vi "SubModule.vi"() -> ()   [LabVIEW 2020]
uses:
  <userlib>/_NEVSTOP/JKI State Machine++/_Support/JKISMQ/_Obtain JKISMQ.vi
  <userlib>/_NEVSTOP/JKI State Machine++/_Support/FGV-BroadcastRegistry/Cache-Broadcast Registry Search Result.vi
  <userlib>/_NEVSTOP/JKI State Machine++/_Support/JKISMQ/_Create Resp Queue.vi
  <userlib>/_NEVSTOP/JKI State Machine++/_Support/JKISMQ/_Unlock JKISMQ.vi
  <userlib>/_NEVSTOP/JKI State Machine++/_Support/JKISMQ/_Lock State JKISMQ.vi
  <userlib>/_NEVSTOP/JKI State Machine++/_Support/JKISMQ/_Release JKISMQ.vi
  <userlib>/_NEVSTOP/JKI State Machine++/_Support/JKISMQ/_Input Name to JKISM Mode.vi
  <userlib>/_NEVSTOP/JKI State Machine++/Utility/uuid.vi
  <userlib>/_NEVSTOP/JKI State Machine++/_Support/FGV-BroadcastRegistry/global-JKISMQ FGV Change Flag.vi
  <userlib>/_NEVSTOP/JKI State Machine++/_Support/JKISMQ/_JKISMQFGV.vi
  <userlib>/_NEVSTOP/JKI State Machine++/_Support/GlobalEvent/FGV-GlobalEventRef.vi
  <userlib>/_NEVSTOP/JKI State Machine++/_Support/JKISMQ/_Dequeue JKISMQ.vi
  <userlib>/_NEVSTOP/JKI State Machine++/_Support/JKISMQ/_Enqueue JKISMQ.vi
  <userlib>/_NEVSTOP/JKI State Machine++/_Support/FGV-BroadcastRegistry/global-Broadcast Cache Change Flag.vi
  <userlib>/_NEVSTOP/JKI State Machine++/_Support/FGV-BroadcastRegistry/FGV-BroadcastRegistry.vi
  <userlib>/_NEVSTOP/JKI State Machine++/JKI State Machine++.lvlib
panel:
  out "State History":string
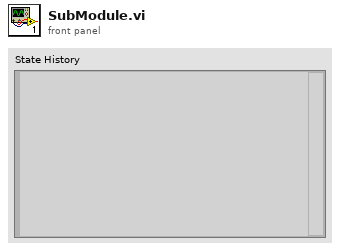
[diagram p1: front panel]
types:
  T1 = enum32{"Invalid", "Standard", "Closed", "Hidden", "Minimized", "Maximized"}
  T2 = enum32{"invalid app kind", "Development System", "Run Time System", "Student Edition", "Embedded LabVIEW", "Evaluation", "Custom"}
  T3 = cluster{"Core":cluster{"Current VI Reference":refnum<vi>, "Close Panel on Exit?":bool}, "Your Boolean data":bool, "Your string data":string}
  T4 = cluster{"Current VI Reference":refnum<vi>, "Close Panel on Exit?":bool}
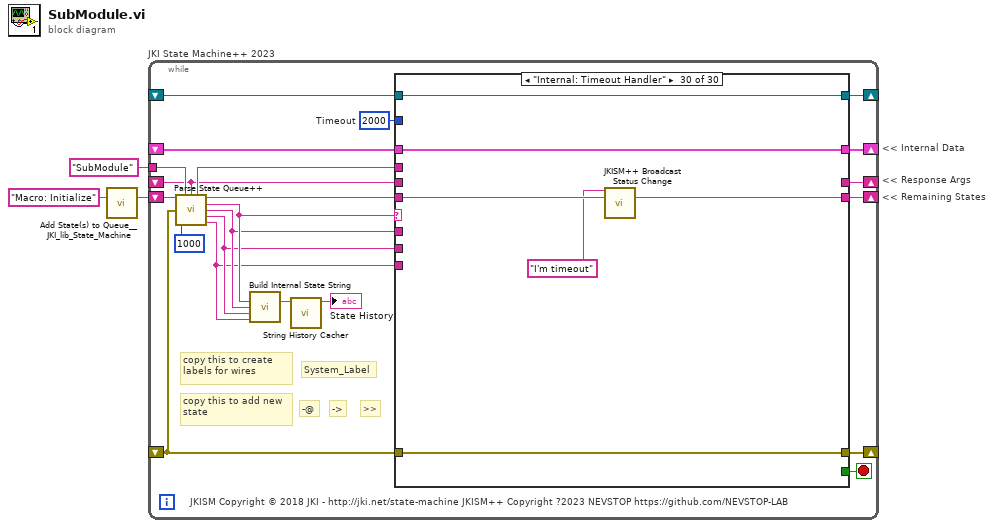
[diagram p0: block diagram]
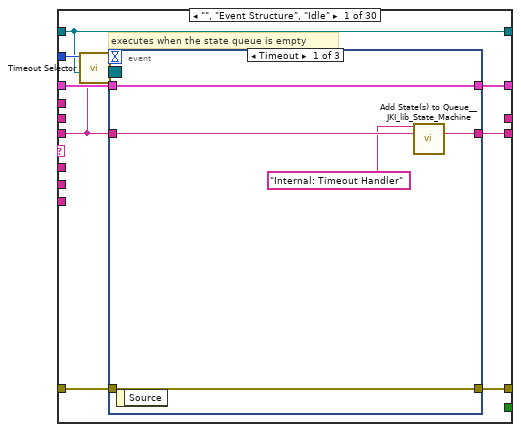
[diagram p2: hidden frame]
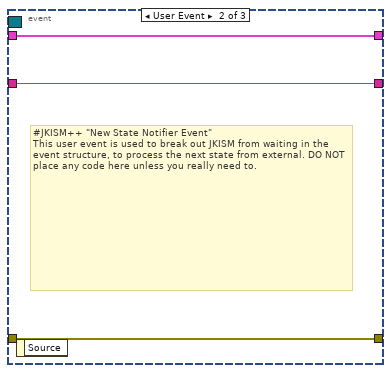
[diagram p3: hidden frame]
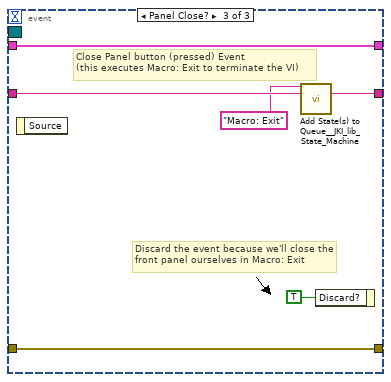
[diagram p4: hidden frame]
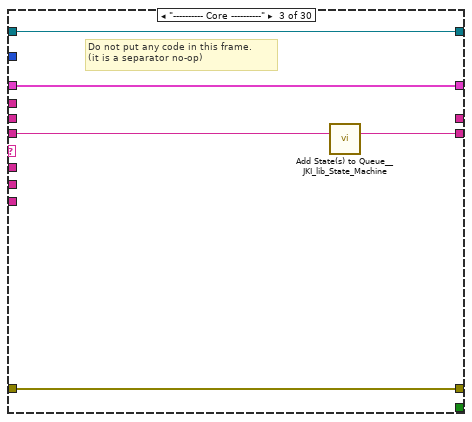
[diagram p6: hidden frame]
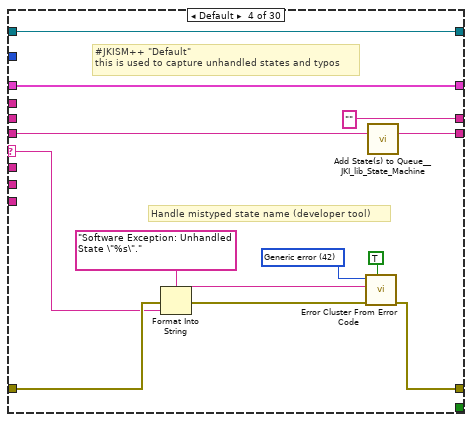
[diagram p7: hidden frame]
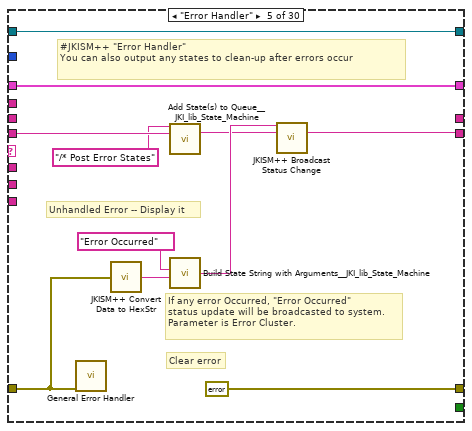
[diagram p8: hidden frame]
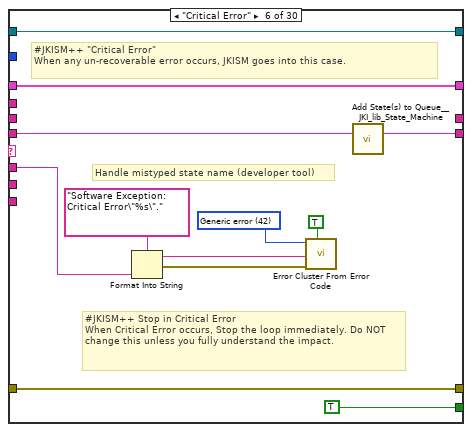
[diagram p9: hidden frame]
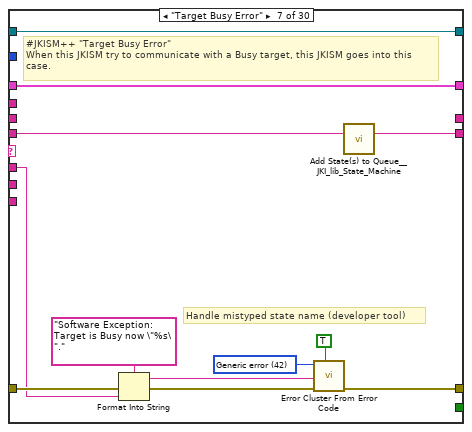
[diagram p10: hidden frame]
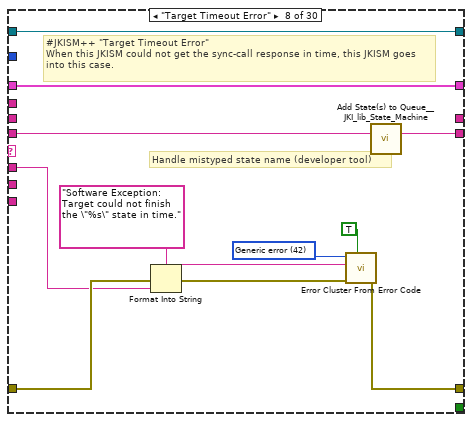
[diagram p11: hidden frame]
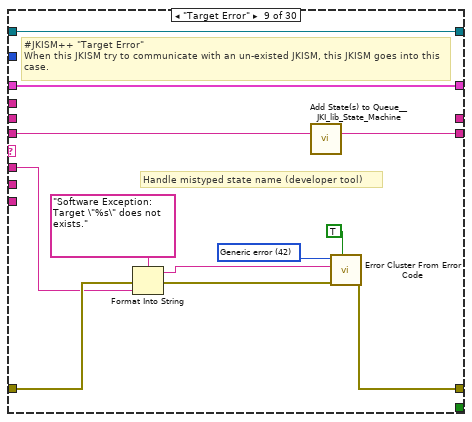
[diagram p12: hidden frame]
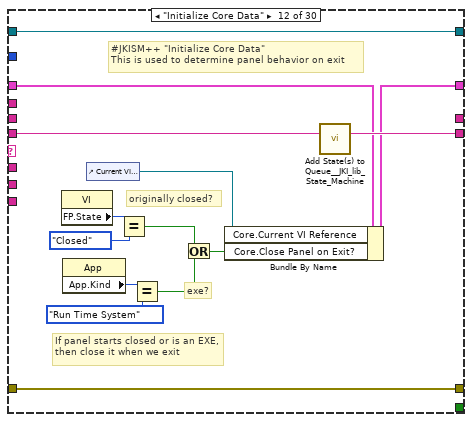
[diagram p15: hidden frame]
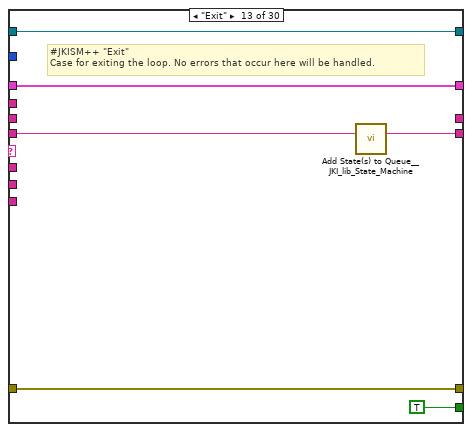
[diagram p16: hidden frame]
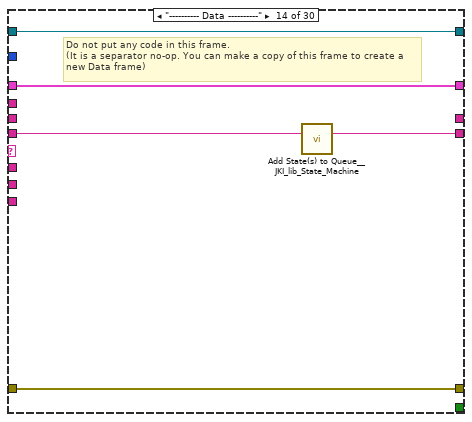
[diagram p17: hidden frame]
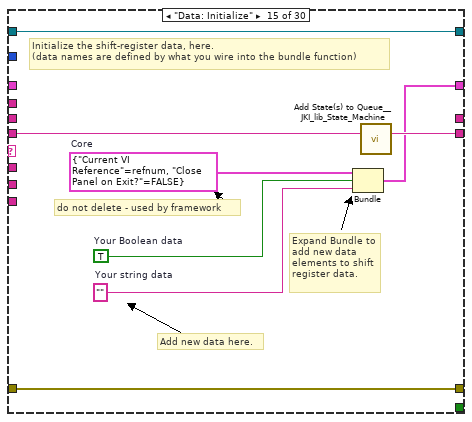
[diagram p18: hidden frame]
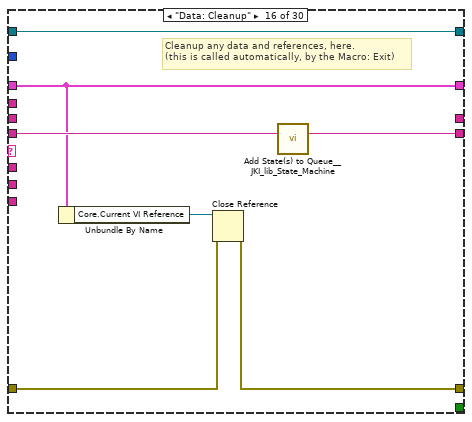
[diagram p19: hidden frame]
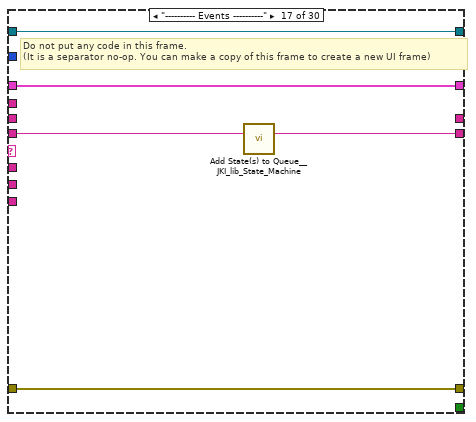
[diagram p20: hidden frame]
diagram:
  # "<< Internal Data"
  # "<< Response Args"
  # "<< Remaining States"
  n1 = call <vilib>:"Add State(s) to Queue__JKI_lib_State_Machine.vi"("State(s) in (\"\")"="Macro: Initialize") -> ("States Out"=w1:string)  [unwired: 14 in]
  n2 = while "JKI State Machine++ 2023" {
    shift-right: [w20] -> _
    shift-left: _ -> [w19]
    shift-right: [w23] -> _
    shift-left: _ -> [w17]
    shift-right: [w22] -> _
    shift-left: w1 -> [w24]
    tunnel: "SubModule" ("Name(\"\" to use uuid)") -> [w12]
    shift-right: [w15] -> _
    shift-left: _ -> [w4]
    shift-right: [w14] -> _
    shift-left: _ -> [w13]
    stop <- w21 stop-if-true
    w18 = 2000  # Timeout
    # "JKISM Copyright © 2018 JKI - http://jki.net/state-machine JKISM++ Copyright ?2023 NEVSTOP https://github.com/NEVSTOP-LAB"
    # "copy this to add new state"
    # ">>"
    # "->"
    # "-@"
    # "copy this to create labels for wires"
    # "System_Label"
    n3 = call <userlib>:"Parse State Queue++.vi"("State Queue"=w24, "Name(\"\" to use uuid)"=w12, "Response Arguments"=w4, "Error In (no error)"=w17, "Response Timeout(5000ms)"=1000 ("Response Timeout(1000ms)")) -> ("Name Used"=w5:string, "Remaining States"=w25:string, "Current State"=w9:string, "Arguments"=w8:string, "Argument - State"=w7:string, "From Who"=w6:string)  [unwired: 5 in]
    n4 = call <userlib>:"Build Internal State String.vi"("State"=w9, "Arguments (\"\")"=w8, "Arg-State (\"\")"=w7, "Source (\"\")"=w6) -> ("State with Arguments"=w10:string)  [unwired: 11 in]
    n5 = call <userlib>:"String History Cacher.vi"("String"=w10) -> ("String Cache"=→"State History":string)  [unwired: 10 in]
    n6 = case shown="\"Internal: Timeout Handler\"" w9 {
      selector: w9 -> [_ _ _ w60 _ _ _ _ _ _ _ _ _ _ _ _ _ _ _ _ _ _ _ _ _ _ _ _ _ _]
      tunnel: w25 -> [w26 w51 w57 w64 w81 w91 w94 w111 w123 w132 w136 w151 w157 w162 w170 w177 w182 w189 w193 w199 w204 w211 w227 w297 w303 w314 w317 w324 w328 w331]
      tunnel: w8 -> [_ _ _ _ _ w84 w96 w107 w119 _ _ _ _ _ _ _ _ _ _ _ _ w206 w221 _ _ _ _ w319 _ _]
      tunnel: w19 -> [w33 w50 w54 w62 w79 w92 w98 w109 w121 w131 w135 w144 w155 w159 _ w172 w179 w188 w192 w196 w202 w209 w223 w294 w300 w311 w316 w323 w327 w334]
      tunnel: [w32 w52 w55 w66 errorcluster {"status"=FALSE, "code"=0, "source"=""} ("error out") w93 w101 w113 w125 w133 w137 w148 w154 w160 w167 w173 w180 w183 w191 w197 w201 w207 w224 w295 w301 w312 w318 w325 w329 w335] -> w23
      tunnel: w17 -> [w31 w52 w55 w65 w71 w93 w100 w112 w124 w133 w137 w148 w154 w160 w167 w174 w180 _ w194 w197 w201 w208 w225 w295 w301 w312 w318 w325 w329 w335]
      tunnel: [w34 w51 w56 w63 w72 w90 w99 w110 w122 w132 w136 w150 w156 w161 w169 w176 w181 w189 w193 w198 w203 w210 w226 w296 w302 w313 w317 w324 w328 w332] -> w22
      tunnel: [_ _ _ _ _ TRUE _ _ _ _ _ _ TRUE _ _ _ _ _ _ _ _ _ _ _ _ _ _ _ _ _] -> w21
      tunnel: [w30 w50 w54 w62 w79 w92 w98 w109 w121 w131 w135 w149 w155 w159 w168 w172 w179 w188 w192 w196 w202 w209 w223 w294 w300 w311 w316 w323 w327 w334] -> w20
      tunnel: w18 -> [w29 _ _ _ _ _ _ _ _ _ _ _ _ _ _ _ _ _ _ _ _ _ _ _ _ _ _ _ _ _]
      tunnel: w6 -> [_ _ _ _ _ _ _ _ _ _ _ _ _ _ _ _ _ _ _ _ _ _ _ _ _ _ _ _ _ _]
      tunnel: w7 -> [_ _ _ _ _ _ _ _ _ _ _ _ _ _ _ _ _ _ _ _ _ _ _ _ _ _ _ _ _ _]
      tunnel: [_ _ _ "" _ _ _ _ _ _ _ _ _ _ _ _ _ _ _ _ _ _ _ _ _ _ _ w320 _ _] -> w15
      tunnel: [w28 w49 w53 w58 w77 w82 w95 w106 w118 w130 w134 w138 w152 w158 w163 w171 w178 w187 w190 w195 w200 w205 w220 w293 w298 w304 w315 w322 w326 w333] -> w14
      tunnel: w13 -> [w28 w49 w53 w58 w77 w82 w95 w106 w118 w130 w134 w138 w152 w158 w163 w171 w178 _ w190 w195 w200 w205 w220 w293 w298 w304 w315 w322 w326 w333]
      tunnel: w5 -> [_ _ _ _ _ _ _ _ _ _ _ _ _ _ _ _ _ w186 _ _ _ _ _ _ _ _ _ _ _ _]
      tunnel: w4 -> [_ _ _ _ _ _ _ _ _ _ _ _ _ _ _ _ _ _ _ _ _ _ _ _ _ _ _ _ _ _]
      frame "", "Event Structure", "Idle" {
        # "executes when the state queue is empty"
        n7 = call <userlib>:"Timeout Selector.vi"("Remaining States"=w26, "Timeout Expected"=w29) -> ("Timeout"=w27:i32)  [unwired: 5 in]
        n8 = event shown="[0] Timeout" {
          selector: w28 -> [_ _ _]
          dyn-events: _ -> [_ _ _]
          timeout: w27 -> [_ _ _]
          tunnel: w26 -> [w39 w41 w48]
          tunnel: [w38 w41 w47] -> w34
          tunnel: w33 -> [w36 w42 w45]
          tunnel: [w37 w40 w46] -> w32
          tunnel: w31 -> [w37 w40 w46]
          tunnel: [w36 w42 w45] -> w30
          event Timeout {
            n9 = event-data() -> ()  [unwired: 1 in, 1 out]
            n10 = call <vilib>:"Add State(s) to Queue__JKI_lib_State_Machine.vi"("State(s) in Front (\"\")"="Internal: Timeout Handler" ("State(s) in Front (\"\")"), "State(s) in (\"\")"=w39) -> ("States Out"=w38:string)  [unwired: 13 in]
          }
          event User Event {
            # "#JKISM++ \"New State Notifier Event\"\nThis user event is used to break out JKISM from waiting in the event structure, to process the next state from external. DO NOT place any code here unless you really need to."
            n11 = event-data() -> ()  [unwired: 1 in, 1 out]
          }
          event Panel Close? {
            # "Discard the event because we'll close the front panel ourselves in Macro: Exit"
            # "Close Panel button (pressed) Event\n(this executes Macro: Exit to terminate the VI)"
            n12 = event-data() -> ()  [unwired: 1 in, 1 out]
            n13 = call <vilib>:"Add State(s) to Queue__JKI_lib_State_Machine.vi"("State(s) in Front (\"\")"="Macro: Exit", "State(s) in (\"\")"=w48) -> ("States Out"=w47:string)  [unwired: 13 in]
            n14 = event-data("Discard?"=TRUE) -> ()  [unwired: 1 in, 1 out]
          }
        }
      }
      frame "JKISM++ Documentation" {
        # "#JKISM++ \"Documentation\"\nCase for holding JKISM++ Documenation"
      }
      frame "---------- Core ----------" {
        # "Do not put any code in this frame.\n(it is a separator no-op)"
        n15 = call <vilib>:"Add State(s) to Queue__JKI_lib_State_Machine.vi"("State(s) in (\"\")"=w57) -> ("States Out"=w56:string)  [unwired: 14 in]
      }
      frame Default {
        w69 = 42 items=["No error", "Argument error", "Memory is full", "Out of zone", "End of file", "File already open", "Generic file I/O error", "File not found", "File permission error", "Disk is full", "Duplicate path", "Too many files open", "System feature not enabled", "Resource file not found", "Cannot add resource", "Resource not found", "Image not found", "Image memory error", "Pen does not exist", "Config type invalid", "Config token not found", "Config parse error", "Config memory error", "Bad external code format", "Bad external code offset", "External code not present", "Null window", "Destroy window error", "Null menu", "Print aborted", "Bad print record", "Print driver error", "Windows error during printing", "Memory error during printing", "Print dialog error", "Generic print error", "Invalid device refnum", "Device not found", "Device parameter error", "Device unit error", "Cannot open device", "Device call aborted", "Generic error", "Cancelled by user", "Object ID too low", "Object ID too high", "Object not in heap", "Unknown heap", "Unknown object (invalid DefProc)", "Unknown object (DefProc not in table)", "Message out of range", "Invalid (null) method", "Unknown message", "Manager call not supported", "Bad address", "Network operation in progress", "Network operation timed out", "Connection is busy", "Network attribute not supported", "Network error", "Address in use", "System out of memory", "Connection aborted", "Connection refused", "Not connected", "Already connected", "Connection closed", "Initialization error (interapplication manager)", "Bad occurrence", "Wait on unbound occurrence handler", "Occurrence queue overflow", "Datalog type conflict", "Unused", "Unrecognized type (interapplication manager)", "Memory corrupt", "Failed to make temporary DLL", "Old CIN version", "Drag socket not found", "Failed to load drop-object", "Failed to register OLE object", "Failed to release OLE object", "Format specifier type mismatch", "Unknown format specifier", "Too few format specifiers", "Too many format specifiers", "Scan failed", "Newer CIN version", "Error converting to variant", "Runtime menu error", "Password tampered", "Variant attribute not found", "Incompatible variant data type", "Event data is not available", "Event Store is not present", "Occurrence is not found", "Event Queue is not created", "Event info is not available", "Refnum passed is NULL", "Error retrieving Class GUID", "Error retrieving CoClass GUID", "Error retrieving TypeLib GUID.", "Bad built application magic bytes.", "Specific driver is different from the specific driver associated with the Logical Name.", "There is no session opened to the class driver.", "Max Error", "MAX - Error with config objects", "MAX - Error loading configuration", "MAX - Group not supported"]
        # "#JKISM++ \"Default\"\nthis is used to capture unhandled states and typos"
        # "Handle mistyped state name (developer tool)"
        n16 = Format Into String(format string="Software Exception: Unhandled State \"%s\"." ("message"), error in=w65, w60) -> (resulting string=w68:string, error out=w67:errorcluster)  [unwired: 1 in]
        n17 = call <vilib>:"Error Cluster From Error Code.vi"("show call chain? (False)"=TRUE, "error in (no error)"=w67, "error message (\"\")"=w68, "error code (0)"=w69) -> ("error out"=w66:errorcluster)  [unwired: 5 in]
        n18 = call <vilib>:"Add State(s) to Queue__JKI_lib_State_Machine.vi"("State(s) in (\"\")"=w64) -> ("States Out"=w63:string)  [unwired: 14 in]
      }
      frame "Error Handler" {
        # "#JKISM++ \"Error Handler\"\nYou can also output any states to clean-up after errors occur"
        # "If any error Occurred, \"Error Occurred\" \nstatus update will be broadcasted to system.\nParameter is Error Cluster."
        # "Unhandled Error -- Display it"
        # "Clear error"
        n19 = call <vilib>:"General Error Handler.vi"("error in (no error)"=w71) -> ()  [unwired: 10 in, 5 out]
        n20 = call <userlib>:"JKISM++ Convert Data to HexStr.vi"("Variant"=w71) -> ("HEX String (0-9,A-F)"=w75:string)  [unwired: 8 in]
        n21 = call <vilib>:"Add State(s) to Queue__JKI_lib_State_Machine.vi"("State(s) in Front (\"\")"="/* Post Error States", "State(s) in (\"\")"=w81) -> ("States Out"=w73:string)  [unwired: 13 in]
        n22 = call <vilib>:"Build State String with Arguments__JKI_lib_State_Machine.vi"("Arguments (\"\")"=w75, "State"="Error Occurred" ("Status with Arguments")) -> ("State with Arguments"=w74:string)  [unwired: 4 in]
        n23 = call <userlib>:"JKISM++ Broadcast Status Change.vi"("Status with Arguments"=w74, "State Queue"=w73) -> ("Remaining States"=w72:string)  [unwired: 13 in]
      }
      frame "Critical Error" {
        w88 = 42 items=["No error", "Argument error", "Memory is full", "Out of zone", "End of file", "File already open", "Generic file I/O error", "File not found", "File permission error", "Disk is full", "Duplicate path", "Too many files open", "System feature not enabled", "Resource file not found", "Cannot add resource", "Resource not found", "Image not found", "Image memory error", "Pen does not exist", "Config type invalid", "Config token not found", "Config parse error", "Config memory error", "Bad external code format", "Bad external code offset", "External code not present", "Null window", "Destroy window error", "Null menu", "Print aborted", "Bad print record", "Print driver error", "Windows error during printing", "Memory error during printing", "Print dialog error", "Generic print error", "Invalid device refnum", "Device not found", "Device parameter error", "Device unit error", "Cannot open device", "Device call aborted", "Generic error", "Cancelled by user", "Object ID too low", "Object ID too high", "Object not in heap", "Unknown heap", "Unknown object (invalid DefProc)", "Unknown object (DefProc not in table)", "Message out of range", "Invalid (null) method", "Unknown message", "Manager call not supported", "Bad address", "Network operation in progress", "Network operation timed out", "Connection is busy", "Network attribute not supported", "Network error", "Address in use", "System out of memory", "Connection aborted", "Connection refused", "Not connected", "Already connected", "Connection closed", "Initialization error (interapplication manager)", "Bad occurrence", "Wait on unbound occurrence handler", "Occurrence queue overflow", "Datalog type conflict", "Unused", "Unrecognized type (interapplication manager)", "Memory corrupt", "Failed to make temporary DLL", "Old CIN version", "Drag socket not found", "Failed to load drop-object", "Failed to register OLE object", "Failed to release OLE object", "Format specifier type mismatch", "Unknown format specifier", "Too few format specifiers", "Too many format specifiers", "Scan failed", "Newer CIN version", "Error converting to variant", "Runtime menu error", "Password tampered", "Variant attribute not found", "Incompatible variant data type", "Event data is not available", "Event Store is not present", "Occurrence is not found", "Event Queue is not created", "Event info is not available", "Refnum passed is NULL", "Error retrieving Class GUID", "Error retrieving CoClass GUID", "Error retrieving TypeLib GUID.", "Bad built application magic bytes.", "Specific driver is different from the specific driver associated with the Logical Name.", "There is no session opened to the class driver.", "Max Error", "MAX - Error with config objects", "MAX - Error loading configuration", "MAX - Group not supported"]
        # "#JKISM++ Stop in Critical Error\nWhen Critical Error occurs, Stop the loop immediately. Do NOT change this unless you fully understand the impact."
        # "#JKISM++ \"Critical Error\"\nWhen any un-recoverable error occurs, JKISM goes into this case."
        # "Handle mistyped state name (developer tool)"
        n24 = Format Into String(format string="Software Exception: Critical Error\"%s\"." ("message"), w84) -> (resulting string=w87:string, error out=w86:errorcluster)  [unwired: 2 in]
        n25 = call <vilib>:"Error Cluster From Error Code.vi"("show call chain? (False)"=TRUE, "error in (no error)"=w86, "error message (\"\")"=w87, "error code (0)"=w88) -> ()  [unwired: 5 in, 1 out]
        n26 = call <vilib>:"Add State(s) to Queue__JKI_lib_State_Machine.vi"("State(s) in (\"\")"=w91) -> ("States Out"=w90:string)  [unwired: 14 in]
      }
      frame "Target Busy Error" {
        w104 = 42 items=["No error", "Argument error", "Memory is full", "Out of zone", "End of file", "File already open", "Generic file I/O error", "File not found", "File permission error", "Disk is full", "Duplicate path", "Too many files open", "System feature not enabled", "Resource file not found", "Cannot add resource", "Resource not found", "Image not found", "Image memory error", "Pen does not exist", "Config type invalid", "Config token not found", "Config parse error", "Config memory error", "Bad external code format", "Bad external code offset", "External code not present", "Null window", "Destroy window error", "Null menu", "Print aborted", "Bad print record", "Print driver error", "Windows error during printing", "Memory error during printing", "Print dialog error", "Generic print error", "Invalid device refnum", "Device not found", "Device parameter error", "Device unit error", "Cannot open device", "Device call aborted", "Generic error", "Cancelled by user", "Object ID too low", "Object ID too high", "Object not in heap", "Unknown heap", "Unknown object (invalid DefProc)", "Unknown object (DefProc not in table)", "Message out of range", "Invalid (null) method", "Unknown message", "Manager call not supported", "Bad address", "Network operation in progress", "Network operation timed out", "Connection is busy", "Network attribute not supported", "Network error", "Address in use", "System out of memory", "Connection aborted", "Connection refused", "Not connected", "Already connected", "Connection closed", "Initialization error (interapplication manager)", "Bad occurrence", "Wait on unbound occurrence handler", "Occurrence queue overflow", "Datalog type conflict", "Unused", "Unrecognized type (interapplication manager)", "Memory corrupt", "Failed to make temporary DLL", "Old CIN version", "Drag socket not found", "Failed to load drop-object", "Failed to register OLE object", "Failed to release OLE object", "Format specifier type mismatch", "Unknown format specifier", "Too few format specifiers", "Too many format specifiers", "Scan failed", "Newer CIN version", "Error converting to variant", "Runtime menu error", "Password tampered", "Variant attribute not found", "Incompatible variant data type", "Event data is not available", "Event Store is not present", "Occurrence is not found", "Event Queue is not created", "Event info is not available", "Refnum passed is NULL", "Error retrieving Class GUID", "Error retrieving CoClass GUID", "Error retrieving TypeLib GUID.", "Bad built application magic bytes.", "Specific driver is different from the specific driver associated with the Logical Name.", "There is no session opened to the class driver.", "Max Error", "MAX - Error with config objects", "MAX - Error loading configuration", "MAX - Group not supported"]
        # "#JKISM++ \"Target Busy Error\"\nWhen this JKISM try to communicate with a Busy target, this JKISM goes into this case."
        # "Handle mistyped state name (developer tool)"
        n27 = Format Into String(format string="Software Exception: Target is Busy now \"%s\"." ("message"), error in=w100, w96) -> (resulting string=w103:string, error out=w102:errorcluster)  [unwired: 1 in]
        n28 = call <vilib>:"Error Cluster From Error Code.vi"("show call chain? (False)"=TRUE, "error in (no error)"=w102, "error message (\"\")"=w103, "error code (0)"=w104) -> ("error out"=w101:errorcluster)  [unwired: 5 in]
        n29 = call <vilib>:"Add State(s) to Queue__JKI_lib_State_Machine.vi"("State(s) in (\"\")"=w94) -> ("States Out"=w99:string)  [unwired: 14 in]
      }
      frame "Target Timeout Error" {
        w116 = 42 items=["No error", "Argument error", "Memory is full", "Out of zone", "End of file", "File already open", "Generic file I/O error", "File not found", "File permission error", "Disk is full", "Duplicate path", "Too many files open", "System feature not enabled", "Resource file not found", "Cannot add resource", "Resource not found", "Image not found", "Image memory error", "Pen does not exist", "Config type invalid", "Config token not found", "Config parse error", "Config memory error", "Bad external code format", "Bad external code offset", "External code not present", "Null window", "Destroy window error", "Null menu", "Print aborted", "Bad print record", "Print driver error", "Windows error during printing", "Memory error during printing", "Print dialog error", "Generic print error", "Invalid device refnum", "Device not found", "Device parameter error", "Device unit error", "Cannot open device", "Device call aborted", "Generic error", "Cancelled by user", "Object ID too low", "Object ID too high", "Object not in heap", "Unknown heap", "Unknown object (invalid DefProc)", "Unknown object (DefProc not in table)", "Message out of range", "Invalid (null) method", "Unknown message", "Manager call not supported", "Bad address", "Network operation in progress", "Network operation timed out", "Connection is busy", "Network attribute not supported", "Network error", "Address in use", "System out of memory", "Connection aborted", "Connection refused", "Not connected", "Already connected", "Connection closed", "Initialization error (interapplication manager)", "Bad occurrence", "Wait on unbound occurrence handler", "Occurrence queue overflow", "Datalog type conflict", "Unused", "Unrecognized type (interapplication manager)", "Memory corrupt", "Failed to make temporary DLL", "Old CIN version", "Drag socket not found", "Failed to load drop-object", "Failed to register OLE object", "Failed to release OLE object", "Format specifier type mismatch", "Unknown format specifier", "Too few format specifiers", "Too many format specifiers", "Scan failed", "Newer CIN version", "Error converting to variant", "Runtime menu error", "Password tampered", "Variant attribute not found", "Incompatible variant data type", "Event data is not available", "Event Store is not present", "Occurrence is not found", "Event Queue is not created", "Event info is not available", "Refnum passed is NULL", "Error retrieving Class GUID", "Error retrieving CoClass GUID", "Error retrieving TypeLib GUID.", "Bad built application magic bytes.", "Specific driver is different from the specific driver associated with the Logical Name.", "There is no session opened to the class driver.", "Max Error", "MAX - Error with config objects", "MAX - Error loading configuration", "MAX - Group not supported"]
        # "#JKISM++ \"Target Timeout Error\"\nWhen this JKISM could not get the sync-call response in time, this JKISM goes into this case."
        # "Handle mistyped state name (developer tool)"
        n30 = Format Into String(format string="Software Exception: Target could not finish the \"%s\" state in time." ("message"), error in=w112, w107) -> (resulting string=w115:string, error out=w114:errorcluster)  [unwired: 1 in]
        n31 = call <vilib>:"Error Cluster From Error Code.vi"("show call chain? (False)"=TRUE, "error in (no error)"=w114, "error message (\"\")"=w115, "error code (0)"=w116) -> ("error out"=w113:errorcluster)  [unwired: 5 in]
        n32 = call <vilib>:"Add State(s) to Queue__JKI_lib_State_Machine.vi"("State(s) in (\"\")"=w111) -> ("States Out"=w110:string)  [unwired: 14 in]
      }
      frame "Target Error" {
        w128 = 42 items=["No error", "Argument error", "Memory is full", "Out of zone", "End of file", "File already open", "Generic file I/O error", "File not found", "File permission error", "Disk is full", "Duplicate path", "Too many files open", "System feature not enabled", "Resource file not found", "Cannot add resource", "Resource not found", "Image not found", "Image memory error", "Pen does not exist", "Config type invalid", "Config token not found", "Config parse error", "Config memory error", "Bad external code format", "Bad external code offset", "External code not present", "Null window", "Destroy window error", "Null menu", "Print aborted", "Bad print record", "Print driver error", "Windows error during printing", "Memory error during printing", "Print dialog error", "Generic print error", "Invalid device refnum", "Device not found", "Device parameter error", "Device unit error", "Cannot open device", "Device call aborted", "Generic error", "Cancelled by user", "Object ID too low", "Object ID too high", "Object not in heap", "Unknown heap", "Unknown object (invalid DefProc)", "Unknown object (DefProc not in table)", "Message out of range", "Invalid (null) method", "Unknown message", "Manager call not supported", "Bad address", "Network operation in progress", "Network operation timed out", "Connection is busy", "Network attribute not supported", "Network error", "Address in use", "System out of memory", "Connection aborted", "Connection refused", "Not connected", "Already connected", "Connection closed", "Initialization error (interapplication manager)", "Bad occurrence", "Wait on unbound occurrence handler", "Occurrence queue overflow", "Datalog type conflict", "Unused", "Unrecognized type (interapplication manager)", "Memory corrupt", "Failed to make temporary DLL", "Old CIN version", "Drag socket not found", "Failed to load drop-object", "Failed to register OLE object", "Failed to release OLE object", "Format specifier type mismatch", "Unknown format specifier", "Too few format specifiers", "Too many format specifiers", "Scan failed", "Newer CIN version", "Error converting to variant", "Runtime menu error", "Password tampered", "Variant attribute not found", "Incompatible variant data type", "Event data is not available", "Event Store is not present", "Occurrence is not found", "Event Queue is not created", "Event info is not available", "Refnum passed is NULL", "Error retrieving Class GUID", "Error retrieving CoClass GUID", "Error retrieving TypeLib GUID.", "Bad built application magic bytes.", "Specific driver is different from the specific driver associated with the Logical Name.", "There is no session opened to the class driver.", "Max Error", "MAX - Error with config objects", "MAX - Error loading configuration", "MAX - Group not supported"]
        # "#JKISM++ \"Target Error\"\nWhen this JKISM try to communicate with an un-existed JKISM, this JKISM goes into this case."
        # "Handle mistyped state name (developer tool)"
        n33 = Format Into String(format string="Software Exception: Target \"%s\" does not exists." ("message"), error in=w124, w119) -> (resulting string=w127:string, error out=w126:errorcluster)  [unwired: 1 in]
        n34 = call <vilib>:"Add State(s) to Queue__JKI_lib_State_Machine.vi"("State(s) in (\"\")"=w123) -> ("States Out"=w122:string)  [unwired: 14 in]
        n35 = call <vilib>:"Error Cluster From Error Code.vi"("show call chain? (False)"=TRUE, "error in (no error)"=w126, "error message (\"\")"=w127, "error code (0)"=w128) -> ("error out"=w125:errorcluster)  [unwired: 5 in]
      }
      frame "Async Response", "Response" {
        # "#JKISM++ Response Comments\nAfter Message is executed, JKISM+ goes to this state for receive the response.\n    For Async Message(->), \"Async Response\" is used. This JKISM will goes to \"Async Message Posted\" immediately and receive the \"Async Response\" after the callee finishes the message.\n    For Sync Message(@),  This JKISM will wait until the message is done and immediately goes to \"Response\""
        # "#JKISM++ \"Async Response\"\nHandle Async-call Response (\"Async Response\" for ->)"
        # "#JKISM++ \"Response\"\nHandle Sync-call Response (\"Response\" for -@)"
      }
      frame "Async Message Posted" {
        # "#JKISM++ \"Async Message Posted\"\nAfter Async Message is posted (-> or ->| ), JKISM+ goes to this state for post-action.\nYou can use Argument - State to tell which Async Message is called."
      }
      frame "Initialize Core Data" {
        # "#JKISM++ \"Initialize Core Data\"\nThis is used to determine panel behavior on exit"
        # "originally closed?"
        # "exe?"
        # "If panel starts closed or is an EXE, then close it when we exit"
        n36 = property class="VI"() -> ("FP.State"=w141:T1)  [unwired: 2 in, 2 out]
        n37 = property class="App"() -> ("App.Kind"=w147:T2)  [unwired: 2 in, 2 out]
        n38 = control-ref of="Current VI Reference"() -> (w142:refnum<vi>)
        n39 = Equal?(x=w141, y=T1."Closed" ("Front Panel Window:State")) -> (x = y?=w139:bool)
        n40 = Equal?(x=w147, y=T2."Run Time System" ("Application:Kind")) -> (x = y?=w145:bool)
        n41 = Or(x=w139, y=w145) -> (x .or. y?=w143:bool)
        n42 = Bundle By Name(cluster=w144, "Core.Current VI Reference"=w142, "Core.Close Panel on Exit?"=w143) -> (w149:T3)
        n43 = call <vilib>:"Add State(s) to Queue__JKI_lib_State_Machine.vi"("State(s) in (\"\")"=w151) -> ("States Out"=w150:string)  [unwired: 14 in]
      }
      frame "Exit" {
        # "#JKISM++ \"Exit\"\nCase for exiting the loop. No errors that occur here will be handled."
        n44 = call <vilib>:"Add State(s) to Queue__JKI_lib_State_Machine.vi"("State(s) in (\"\")"=w157) -> ("States Out"=w156:string)  [unwired: 14 in]
      }
      frame "---------- Data ----------" {
        # "Do not put any code in this frame.\n(It is a separator no-op. You can make a copy of this frame to create a new Data frame)"
        n45 = call <vilib>:"Add State(s) to Queue__JKI_lib_State_Machine.vi"("State(s) in (\"\")"=w162) -> ("States Out"=w161:string)  [unwired: 14 in]
      }
      frame "Data: Initialize" {
        w164 = T4 {"Current VI Reference"=refnum, "Close Panel on Exit?"=FALSE}  # Core
        w166 = TRUE  # Your Boolean data
        w165 = ""  # Your string data
        # "do not delete - used by framework"
        # "Expand Bundle to add new data elements to shift register data."
        # "Add new data here."
        # "Initialize the shift-register data, here.\n(data names are defined by what you wire into the bundle function)"
        n46 = Bundle("Core"=w164, "Your Boolean data"=w166, "Your string data"=w165) -> (w168:T3)  [unwired: 1 in]
        n47 = call <vilib>:"Add State(s) to Queue__JKI_lib_State_Machine.vi"("State(s) in (\"\")"=w170) -> ("States Out"=w169:string)  [unwired: 14 in]
      }
      frame "Data: Cleanup" {
        # "Cleanup any data and references, here.\n(this is called automatically, by the Macro: Exit)"
        n48 = Unbundle By Name(w172) -> ("Core.Current VI Reference"=w175:refnum<vi>)
        n49 = Close Reference(reference=w175, error in (no error)=w174) -> (error out=w173:errorcluster)
        n50 = call <vilib>:"Add State(s) to Queue__JKI_lib_State_Machine.vi"("State(s) in (\"\")"=w177) -> ("States Out"=w176:string)  [unwired: 14 in]
      }
      frame "---------- Events ----------" {
        # "Do not put any code in this frame.\n(It is a separator no-op. You can make a copy of this frame to create a new UI frame)"
        n51 = call <vilib>:"Add State(s) to Queue__JKI_lib_State_Machine.vi"("State(s) in (\"\")"=w182) -> ("States Out"=w181:string)  [unwired: 14 in]
      }
      frame "Events: Register" {
        # "#JKISM++ \"Events: Register\"\nRegister user event. New Message Event is registered to break JKISM waiting in event structure by default."
        # "#JKISM++ Register New Message Event\nRegister message event to break Waiting in Event structure."
        n52 = call <userlib>:"JKISM++ Get New State Notifier Event.vi"("Name(\"\" to use uuid) in"=w186) -> ("Error out"=w184:errorcluster, "New State Notifier Event"=w185:refnum<user-event>)  [unwired: 9 in]
        n53 = register-events(error in=w184, w185) -> (reference out=w187:refnum<event-registration>, error out=w183:errorcluster)  [unwired: 1 in]
      }
      frame "Events: Unregister" {
        # "#JKISM++ \"Events: Unregister\"\nUnregister user event."
        n54 = Unregister For Events(event registration refnum=w190, error in=w194) -> (error out=w191:errorcluster)
      }
      frame "---------- UI ----------" {
        # "Do not put any code in this frame.\n(It is a separator no-op. You can make a copy of this frame to create a new UI frame)"
        n55 = call <vilib>:"Add State(s) to Queue__JKI_lib_State_Machine.vi"("State(s) in (\"\")"=w199) -> ("States Out"=w198:string)  [unwired: 14 in]
      }
      frame "UI: Initialize" {
        # "#JKISM++ \"UI: Initialize\"\nInitialize the User Interface, here.\n(this is called automatically, by the Macro: Init)"
        n56 = call <vilib>:"Add State(s) to Queue__JKI_lib_State_Machine.vi"("State(s) in (\"\")"=w204) -> ("States Out"=w203:string)  [unwired: 14 in]
      }
      frame "UI: Cursor Set" {
        # "#JKISM++ \"UI: Cursor Set\"\nSet and Unset Cursor Busy.\n(Usage: \"UI: Cursor Set >> Busy|Idle\")"
        # "Argument"
        n57 = disable-structure shown="Default" {
          disable-tunnel: w208 -> [w214 w219]
          disable-tunnel: [w213 w219] -> w207
          disable-tunnel: w206 -> [w212 _]
          frame condition #0 (active) {
            n58 = case shown="\"Idle\", Default" w212 {
              tunnel: w214 -> [w216 w218]
              tunnel: [w215 w217] -> w213
              frame "Idle", Default {
                n59 = call <vilib>:"Unset Busy.vi"("error in (no error)"=w216) -> ("error out"=w215:errorcluster)  [unwired: 10 in]
              }
              frame "Busy" {
                n60 = call <vilib>:"Set Busy.vi"("error in (no error)"=w218) -> ("error out"=w217:errorcluster)  [unwired: 9 in, 1 out]
              }
            }
          }
          frame condition #1 {
          }
        }
        n61 = call <vilib>:"Add State(s) to Queue__JKI_lib_State_Machine.vi"("State(s) in (\"\")"=w211) -> ("States Out"=w210:string)  [unwired: 14 in]
      }
      frame "UI: Front Panel State" {
        # "#JKISM++ \"UI: Front Panel State\"\nSet Front Panel Open or Closed\n(Usage: \"UI: Front Panel State >> Open|Close\")"
        # "Argument"
        n62 = Unbundle By Name(w223) -> ("Core.Current VI Reference"=w222:refnum<vi>)
        n63 = call <vilib>:"Add State(s) to Queue__JKI_lib_State_Machine.vi"("State(s) in (\"\")"=w227) -> ("States Out"=w226:string)  [unwired: 14 in]
        n64 = case shown="\"Close\", \"Closed\"" w221 {
          tunnel: w225 -> [w233 w248 w259 w272 w285]
          tunnel: [w235 w249 w261 w274 w287] -> w224
          tunnel: w222 -> [w234 w246 w260 w273 w286]
          frame "Open", "Standard", Default {
            w228 = T1."Standard" ("State")
            n65 = property class="VI"(reference=w234, error in=w233) -> (reference out=w231:refnum<vi>, error out=w232:errorcluster, "FP.State"=w230:T1)
            n66 = Not Equal?(x=w230, y=w228) -> (x != y?=w229:bool)
            n67 = case shown="True" w229 {
              tunnel: [w239 w241] -> w235
              tunnel: w232 -> [w238 w241]
              tunnel: w231 -> [w237 _]
              tunnel: w228 -> [w236 _]
              frame True {
                n68 = invoke class="VI" method="FP.Open"(reference=w237, error in=w238, "Activate"=TRUE, "State"=w236) -> (error out=w239:errorcluster)  [unwired: 1 in, 4 out]
              }
              frame False {
              }
            }
          }
          frame "Close", "Closed" {
            n69 = property class="VI"(reference=w246, error in=w248) -> (reference out=w245:refnum<vi>, error out=w247:errorcluster, "FP.State"=w243:T1)
            n70 = Not Equal?(x=w243, y=T1."Closed" ("Front Panel Window:State")) -> (x != y?=w242:bool)
            n71 = case shown="False" w242 {
              tunnel: [w250 w253] -> w249
              tunnel: w247 -> [w250 w252]
              tunnel: w245 -> [_ w251]
              frame False {
              }
              frame True {
                n72 = invoke class="VI" method="FP.Close"(reference=w251, error in=w252) -> (error out=w253:errorcluster)  [unwired: 1 in, 2 out]
              }
            }
          }
          frame "Hidden", "Hide" {
            w254 = T1."Hidden" ("State")
            n73 = property class="VI"(reference=w260, error in=w259) -> (reference out=w257:refnum<vi>, error out=w258:errorcluster, "FP.State"=w256:T1)
            n74 = Not Equal?(x=w256, y=w254) -> (x != y?=w255:bool)
            n75 = case shown="True" w255 {
              tunnel: [w265 w266] -> w261
              tunnel: w258 -> [w264 w266]
              tunnel: w257 -> [w263 _]
              tunnel: w254 -> [w262 _]
              frame True {
                n76 = invoke class="VI" method="FP.Open"(reference=w263, error in=w264, "State"=w262) -> (error out=w265:errorcluster)  [unwired: 2 in, 4 out]
              }
              frame False {
              }
            }
          }
          frame "Minimize", "Minimized" {
            w267 = T1."Minimized" ("State")
            n77 = property class="VI"(reference=w273, error in=w272) -> (reference out=w270:refnum<vi>, error out=w271:errorcluster, "FP.State"=w269:T1)
            n78 = Not Equal?(x=w269, y=w267) -> (x != y?=w268:bool)
            n79 = case shown="True" w268 {
              tunnel: [w278 w279] -> w274
              tunnel: w271 -> [w277 w279]
              tunnel: w270 -> [w276 _]
              tunnel: w267 -> [w275 _]
              frame True {
                n80 = invoke class="VI" method="FP.Open"(reference=w276, error in=w277, "State"=w275) -> (error out=w278:errorcluster)  [unwired: 2 in, 4 out]
              }
              frame False {
              }
            }
          }
          frame "Maximize", "Maximized" {
            w280 = T1."Maximized" ("State")
            n81 = property class="VI"(reference=w286, error in=w285) -> (reference out=w283:refnum<vi>, error out=w284:errorcluster, "FP.State"=w282:T1)
            n82 = Not Equal?(x=w282, y=w280) -> (x != y?=w281:bool)
            n83 = case shown="True" w281 {
              tunnel: [w291 w292] -> w287
              tunnel: w284 -> [w290 w292]
              tunnel: w283 -> [w289 _]
              tunnel: w280 -> [w288 _]
              frame True {
                n84 = invoke class="VI" method="FP.Open"(reference=w289, error in=w290, "State"=w288) -> (error out=w291:errorcluster)  [unwired: 2 in, 4 out]
              }
              frame False {
              }
            }
          }
        }
      }
      frame "---------- Macro ----------" {
        # "Do not put any code in this frame.\n(It is a separator no-op. You can make a copy of this frame to create a new Macro frame)"
        n85 = call <vilib>:"Add State(s) to Queue__JKI_lib_State_Machine.vi"("State(s) in (\"\")"=w297) -> ("States Out"=w296:string)  [unwired: 14 in]
      }
      frame "Macro: Initialize" {
        w299 = "Data: Initialize\nInitialize Core Data\nEvents: Register\nUI: Initialize\nUI: Front Panel State >> Open"  # Data: Initialize Initialize Core Data Events: Register UI: Initialize UI: Front Panel State >> Open
        # "#JKISM++ \"Macro: Initialize\"\nInitialization Macro (This is called once, when the VI starts)"
        n86 = call <vilib>:"Add State(s) to Queue__JKI_lib_State_Machine.vi"("State(s) in Front (\"\")"=w299, "State(s) in (\"\")"=w303) -> ("States Out"=w302:string)  [unwired: 13 in]
      }
      frame "Macro: Exit" {
        # "#JKISM++ \"Macro: Exit\"\nExit Macro (This is called once, when the VI exits)"
        n87 = Unbundle By Name(w311) -> ("Core.Close Panel on Exit?"=w310:bool)
        n88 = Select(t="UI: Front Panel State >> Close", s=w310, f="") -> (s? t:f=w307:string)
        n89 = call <vilib>:"Add State(s) to Queue__JKI_lib_State_Machine.vi"("State(s) in (\"\")"=w307, "State(s) at Back (\"\")"="Data: Cleanup\nEvents: Unregister\nExit") -> ("States Out"=w305:string)  [unwired: 13 in]
        n90 = call <vilib>:"Add State(s) to Queue__JKI_lib_State_Machine.vi"("State(s) in Front (\"\")"=w305, "State(s) in (\"\")"=w314) -> ("States Out"=w313:string)  [unwired: 13 in]
      }
      frame "---------- API ----------" {
        # "Do not put any code in this frame.\n(It is a separator no-op. This category is recommended to use for external API)"
      }
      frame "API: EchoArguments" {
        n91 = Concatenate Strings("Response:", w319) -> (w320:string)
      }
      frame "------ Internal ---------" {
      }
      frame "Internal: Timeout Handler" {
        n92 = call <userlib>:"JKISM++ Broadcast Status Change.vi"("Status with Arguments"="I'm timeout", "State Queue"=w331) -> ("Remaining States"=w332:string)  [unwired: 13 in]
      }
    }
  }
